vi "Manage String Size.vi"(1 "String In":string, 12 "Max String Size":i32) -> (21 "String Out":string)   [LabVIEW 2015]
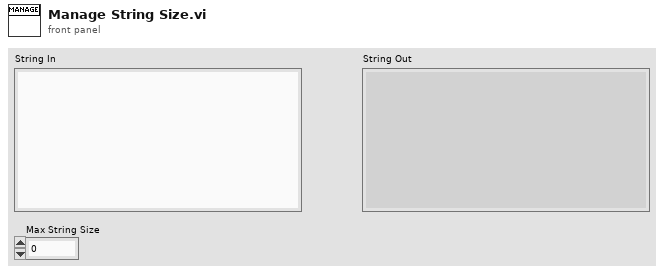
[diagram p1: front panel]
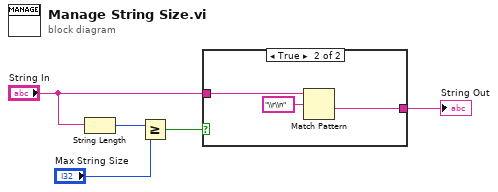
[diagram p0: block diagram]
diagram:
  n1 = String Length(string="String In") -> (length=w5:i32)
  n2 = Greater Or Equal?(x=w5, y="Max String Size") -> (x >= y?=w2:bool)
  n3 = case shown="True" w2 {
    tunnel: "String In" -> [w6 w9]
    tunnel: [w6 w7] -> w1
    frame False {
    }
    frame True {
      n4 = Match Pattern(string=w9, regular expression="\\r\\n") -> (after substring=w7:string)  [unwired: 1 in, 3 out]
    }
  }
  "String Out" <- w1
